vi "Insert Value[] (Boolean).vi"(7 "key":string[](array[string]), 8 "error in (no error)":errorcluster, 10 "JSON Data in":bool, 11 "JSON Value in":refnum<class "JSON Value.lvclass">) -> (0 "error out":errorcluster, 1 "replaced":bool, 3 "JSON Value out":refnum<class "JSON Value.lvclass">)   [LabVIEW 2016, in "JSON Value.lvclass"]
uses:
  JSON Value.lvclass
  New JSON Value/New JSON (Boolean).vi
  Insert Value (Value).vi
  Array/Replace Array Subset/Replace Array Subset (Value).vi
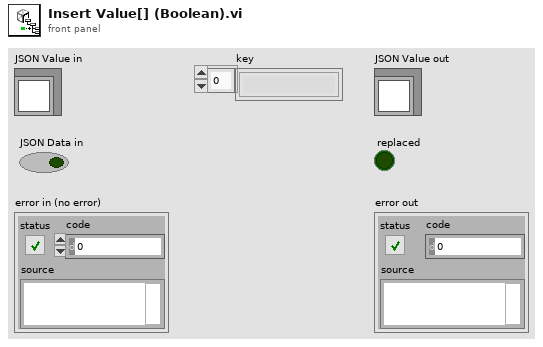
[diagram p1: front panel]
types:
  T1 = typedef "JSON Value.lvclass/JSON Types.ctl" = enum16{"String", "Numeric", "Boolean", "NULL", "Object", "Array"}
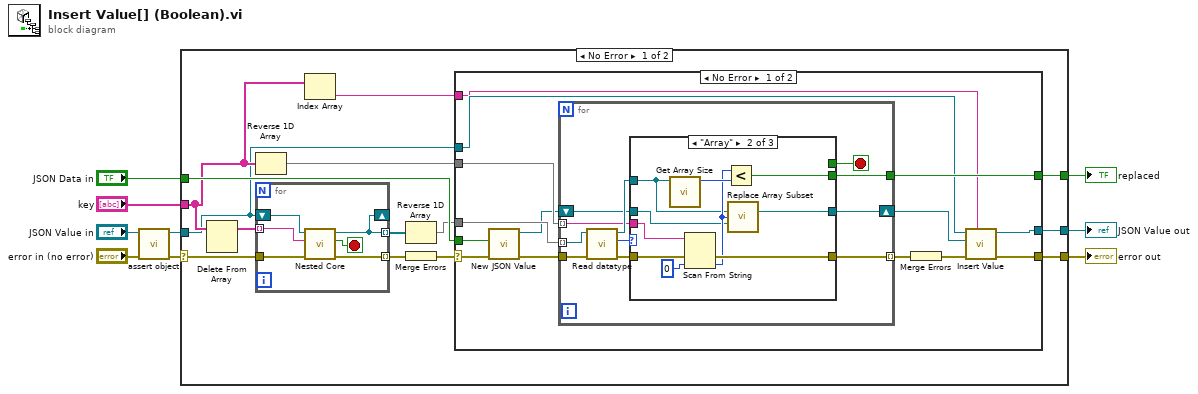
[diagram p0: block diagram]
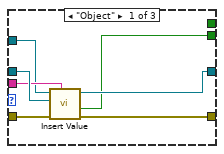
[diagram p2: hidden frame]
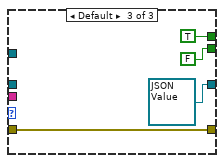
[diagram p3: hidden frame]
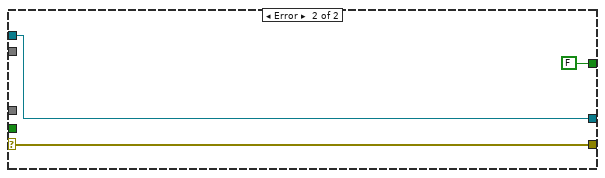
[diagram p4: hidden frame]
diagram:
  n1 = call "assert object.vi"("error in (no error)"="error in (no error)", "JSON Value in"="JSON Value in") -> ("error out"=w3:errorcluster, "JSON Value out"=w1:refnum<class "JSON Value.lvclass">)  [unwired: 8 in]
  n2 = case shown="No Error" w3 {
    selector: w3 -> [w11 w80]
    tunnel: [w23 _] -> w9
    tunnel: "JSON Data in" -> [w22 _]
    tunnel: [w15 w79] -> w6
    tunnel: [w14 w80] -> w5
    tunnel: "key" -> [w13 _]
    tunnel: w1 -> [w10 w79]
    frame No Error {
      n3 = Delete From Array(array=w13) -> (array with subset deleted=w19:string[])  [unwired: 2 in, 1 out]
      n4 = Reverse 1D Array(array=w13) -> (reversed array=w20:string[])
      n5 = for {
        tunnel: w19 -> [w78] mode=indexing
        shift-right: [w73] -> _
        shift-left: w10 -> [w77]
        tunnel: w11 -> [w76]
        tunnel: [w75] -> w16 mode=indexing
        tunnel: [w73] -> w17 mode=indexing
        stop <- w74 stop-if-true
        n6 = call "Nested Core.vi"("error in (no error)"=w76, "key"=w78, "JSON Value in"=w77) -> ("error out"=w75:errorcluster, "stop?"=w74:bool, "JSON Value out"=w73:refnum<class "JSON Value.lvclass">)  [unwired: 6 in]
      }
      n7 = Index Array(array=w13) -> (element=w12:string)  [unwired: 1 in]
      n8 = Reverse 1D Array(array=w17) -> (reversed array=w21:refnum<class "JSON Value.lvclass">[])
      n9 = Merge Errors(w16) -> (w18:errorcluster)
      n10 = case shown="No Error" w18 {
        selector: w18 -> [w25 w70]
        tunnel: [w37 FALSE ("replaced")] -> w23
        tunnel: w22 -> [w27 _]
        tunnel: w21 -> [w36 _]
        tunnel: w20 -> [w35 _]
        tunnel: [w31 w72] -> w15
        tunnel: w10 -> [w33 w72]
        tunnel: [w29 w70] -> w14
        tunnel: w12 -> [w28 _]
        frame No Error {
          n11 = call-poly "New JSON Value.vi"("error in (no error)"=w25, "value"=w27) -> ("error out"=w24:errorcluster, "JSON Value out"=w26:refnum<class "JSON Value.lvclass">)  [unwired: 8 in]
          n12 = for {
            tunnel: w35 -> [w40] mode=indexing
            tunnel: w24 -> [w46]
            tunnel: [w45] -> w34 mode=indexing
            tunnel: [w42] -> w37
            tunnel: w36 -> [w41] mode=indexing
            shift-right: [w39] -> w32
            shift-left: w26 -> [w38]
            stop <- w43 stop-if-true
            n13 = call "Read datatype.vi"("error in (no error)"=w46, "JSON Value in"=w41) -> ("error out"=w44:errorcluster, "datatype"=w47:T1, "JSON Value out"=w48:refnum<class "JSON Value.lvclass">)  [unwired: 7 in]
            n14 = case shown="\"Array\"" w47 {
              tunnel: w40 -> [w51 w60 _]
              tunnel: [w53 w57 refnum<class "JSON Value.lvclass"> refnum ("JSON Object in")] -> w39
              tunnel: w48 -> [w50 w56 _]
              tunnel: [w55 w63 w68] -> w45
              tunnel: w44 -> [w49 w64 w68]
              tunnel: [_ _ TRUE] -> w43
              tunnel: [w52 w61 FALSE] -> w42
              tunnel: w38 -> [w54 w58 _]
              frame "Object" {
                n15 = call-poly "Insert Value.vi"("key"=w51, "error in (no error)"=w49, 10:"JSON Value in"=w54, 11:"JSON Value in"=w50) -> ("error out"=w55:errorcluster, "replaced"=w52:bool, "JSON Value out"=w53:refnum<class "JSON Value.lvclass">)  [unwired: 5 in]
              }
              frame "Array" {
                n16 = call "Get Array Size.vi"("JSON Value in"=w56) -> ("size(s)"=w62:i32)  [unwired: 9 in, 1 out]
                n17 = Scan From String(input string=w60, error in=w64, default 1=0 ("index")) -> (error out=w63:errorcluster, output 1=w59:i32)  [unwired: 2 in, 2 out]
                n18 = Less?(x=w59, y=w62) -> (x < y?=w61:bool)
                n19 = call-poly "Replace Array Subset.vi"("JSON Array"=w56, "index"=w59, "new element/subarray"=w58) -> ("output JSON Array"=w57:refnum<class "JSON Value.lvclass">)  [unwired: 11 in, 1 out]
              }
              frame Default {
              }
            }
          }
          n20 = Merge Errors(w34) -> (w30:errorcluster)
          n21 = call-poly "Insert Value.vi"("key"=w28, "error in (no error)"=w30, 10:"JSON Value in"=w32, 11:"JSON Value in"=w33) -> ("error out"=w29:errorcluster, "JSON Value out"=w31:refnum<class "JSON Value.lvclass">)  [unwired: 5 in, 1 out]
        }
        frame Error {
        }
      }
    }
    frame Error {
    }
  }
  "replaced" <- w9
  "error out" <- w5
  "JSON Value out" <- w6
